vi "sum_Array.vi"(2 "axis":enum16{"None", "0", "1"}(ring), 3 "z":dbl[][](array[numeric])) -> (0 "scalar":dbl, 1 "sum":dbl[][](array[numeric]))   [LabVIEW 2020]
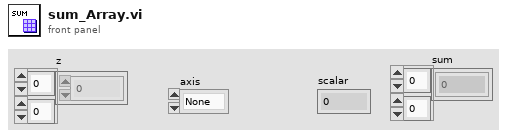
[diagram p1: front panel]
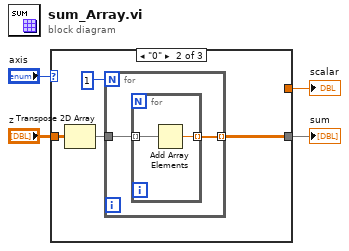
[diagram p0: block diagram]
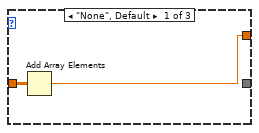
[diagram p2: hidden frame]
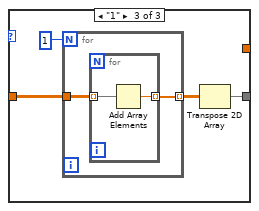
[diagram p3: hidden frame]
diagram:
  n1 = case shown="\"0\"" "axis" {
    tunnel: "z" -> [w6 w10 w16]
    tunnel: [w5 _ _] -> w1
    tunnel: [_ w9 w17] -> w2
    frame "None", Default {
      n2 = Add Array Elements(numeric array=w6) -> (sum=w5:dbl)
    }
    frame "0" {
      n3 = Transpose 2D Array(2D array=w10) -> (transposed array=w7:dbl[][])
      n4 = for {
        N: 1 -> [_]
        tunnel: w7 -> [w12]
        tunnel: [w11] -> w9 mode=indexing
        n5 = for {
          tunnel: w12 -> [w14] mode=indexing
          tunnel: [w13] -> w11 mode=indexing
          n6 = Add Array Elements(numeric array=w14) -> (sum=w13:dbl)
        }
      }
    }
    frame "1" {
      n7 = for {
        N: 1 -> [_]
        tunnel: [w20] -> w18 mode=indexing
        tunnel: w16 -> [w19]
        n8 = for {
          tunnel: [w22] -> w20 mode=indexing
          tunnel: w19 -> [w21] mode=indexing
          n9 = Add Array Elements(numeric array=w21) -> (sum=w22:dbl)
        }
      }
      n10 = Transpose 2D Array(2D array=w18) -> (transposed array=w17:dbl[][])
    }
  }
  "sum" <- w2
  "scalar" <- w1
